vi "Multi Scan Average.vi"(8 "error in (no error)":errorcluster caption="entrée d'erreur (pas d'erreur)") -> (0 "error out":errorcluster caption="sortie d'erreur")   [LabVIEW 2019, in "Calculations.lvclass"]
uses:
  Calculations Class/Calculations.lvclass
  C:/Programmes Labview/LabScanV1A/DevicesClass/BaseDevice/BaseDevice.lvclass
  DevicesClass/BaseDevice/Accessor/GetClassEvent.vi
panel:
  out "Calculations Out.lvclass":refnum<class "Calculations.lvclass">
  in  "Calculations.lvclass":refnum<class "Calculations.lvclass">
  in  "Tab":enum32{"Description"}(tab)
  out "CalcDescription":string="Perform a running average on the selected data source. The function will average the last n data samples, where n is the \"Sample Count\" parameter provided"
  out "CalcPanelName":string="Multi Scan Average"
  in  "EditorProgQ":refnum<queue>
  in  "EditorProgQEvent":refnum<user-event>
  in  "Stop":bool
  out "Init Program":bool
  # "Multi Scan Average"
  # "this MUST be present and labeled \"Stop\""
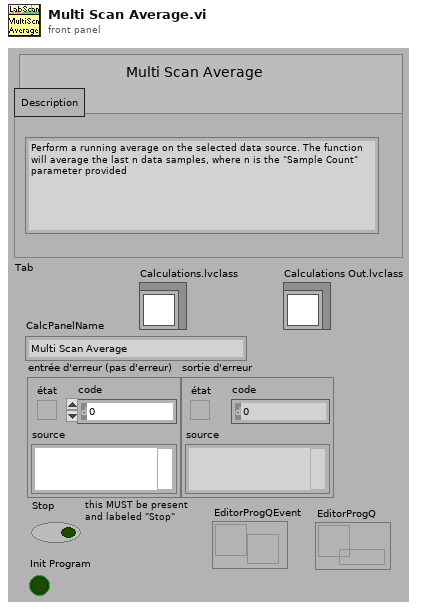
[diagram p1: front panel]
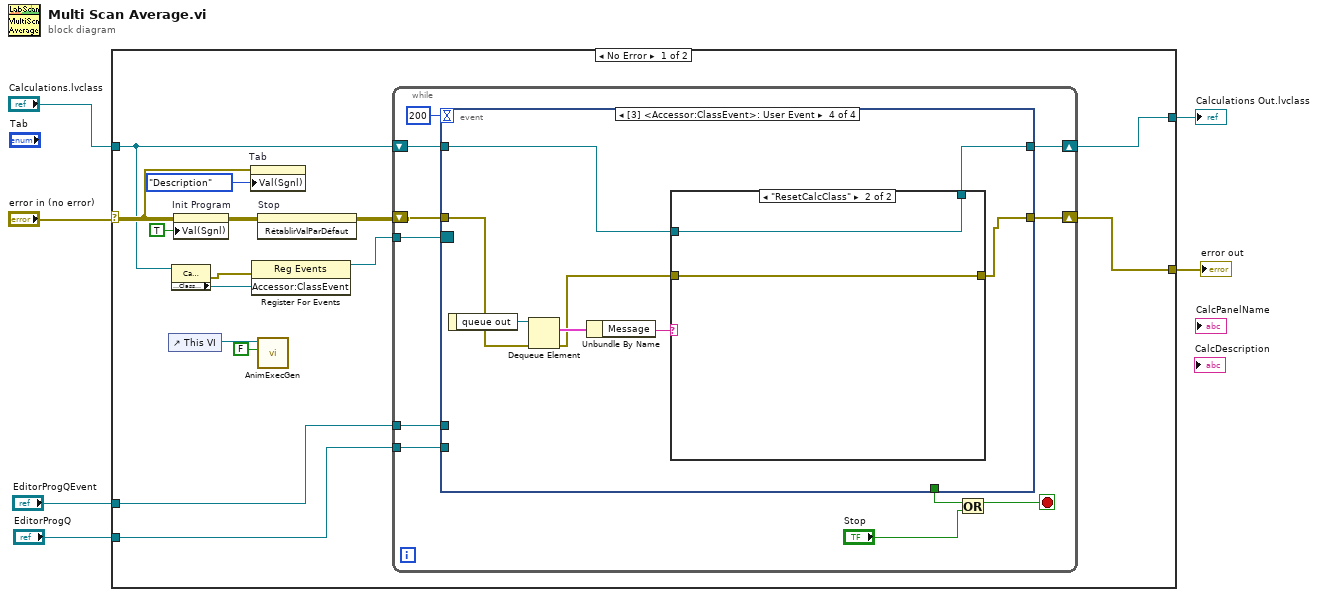
[diagram p0: block diagram]
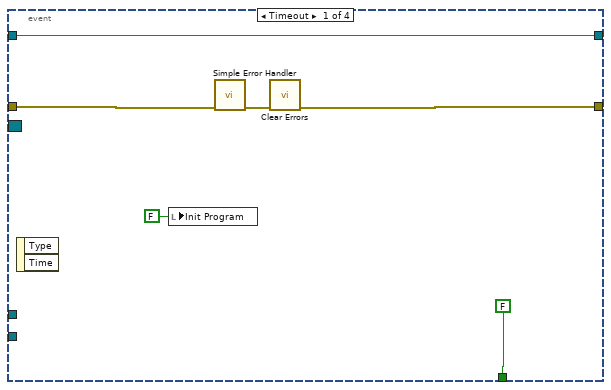
[diagram p2: hidden frame]
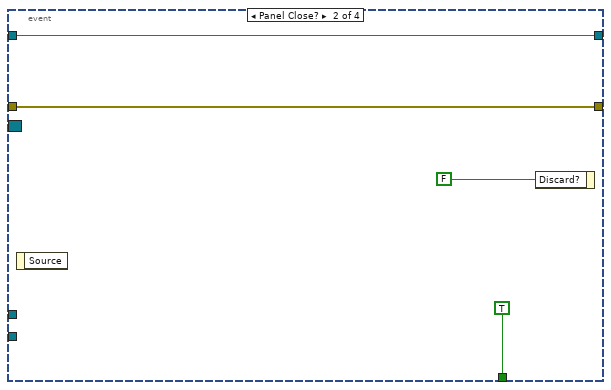
[diagram p3: hidden frame]
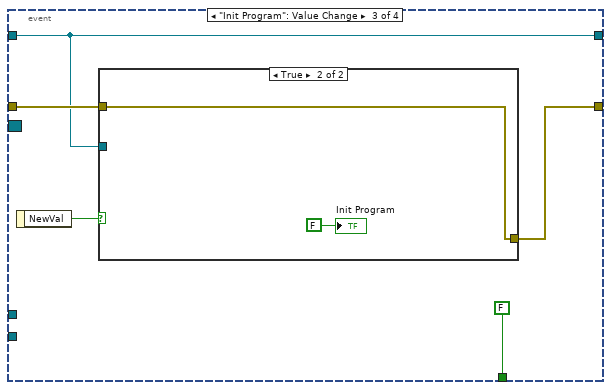
[diagram p4: hidden frame]
diagram:
  n1 = case shown="No Error" "error in (no error)" {
    selector: "error in (no error)" -> [w7 w64]
    tunnel: [w21 w64] -> w5
    tunnel: "EditorProgQEvent" -> [w15 _]
    tunnel: "EditorProgQ" -> [w14 _]
    tunnel: "Calculations.lvclass" -> [w9 w63]
    tunnel: [w13 w63] -> w1
    frame No Error {
      n2 = control-ref of="This VI"() -> (w16:refnum<vi>)
      n3 = property class="Calculations.lvclass"(reference=w9) -> (error out=w12:errorcluster, "Accessor:ClassEvent"=w11:refnum<user-event>)  [unwired: 1 in, 1 out]
      n4 = property on="Init Program" class="Bool (strict)"(error in=w7, "Val(Sgnl)"=TRUE ("Valeur (Signalisation)")) -> (error out=w19:errorcluster)  [unwired: 1 in, 1 out]
      n5 = property on="Tab" class="Onglet (strict)"(error in=w7, "Val(Sgnl)"=enum32{"Description"}."Description" ("Valeur (Signalisation)")) -> ()  [unwired: 1 in, 2 out]
      n6 = register-events(error in=w12, w11) -> (reference out=w10:refnum<event-registration>)  [unwired: 1 in, 1 out]
      n7 = invoke on="Stop" class="Bool (strict)" method="RétablirValParDéfaut"(error in=w19) -> (error out=w18:errorcluster)  [unwired: 2 in, 2 out]
      n8 = call <userlib>:"AnimExecGen.vi"("Animer l'exécution ?"=FALSE, "ViRef"=w16) -> ()  [unwired: 9 in, 1 out]
      n9 = while {
        shift-right: [w30] -> w21
        shift-left: w18 -> [w31]
        tunnel: w15 -> [w26]
        tunnel: w14 -> [w25]
        shift-right: [w23] -> w13
        shift-left: w9 -> [w24]
        tunnel: w10 -> [w22]
        stop <- w28 stop-if-true
        n10 = event shown="[3] <Accessor:ClassEvent>: User Event" {
          selector: w22 -> [_ _ _ _]
          dyn-events: _ -> [_ _ _ _]
          timeout: 200 -> [_ _ _ _]
          tunnel: w31 -> [w37 w40 w46 w52]
          tunnel: [w35 w40 w45 w54] -> w30
          tunnel: [FALSE TRUE FALSE _] -> w29
          tunnel: w26 -> [_ _ _ _]
          tunnel: w25 -> [_ _ _ _]
          tunnel: w24 -> [w33 w39 w43 w55]
          tunnel: [w33 w39 w43 w56] -> w23
          event Timeout {
            n11 = event-data() -> ()  [unwired: 1 in, 2 out]
            n12 = local write "Init Program"(FALSE ("Init Program")) -> ()
            n13 = call <vilib>:"Simple Error Handler.vi"("error in (no error)"=w37) -> ("error out"=w36:errorcluster)  [unwired: 4 in, 4 out]
            n14 = call <vilib>:"Clear Errors.vi"("error in (no error)"=w36) -> ("error out"=w35:errorcluster)  [unwired: 5 in, 1 out]
          }
          event Panel Close? {
            n15 = event-data() -> ()  [unwired: 1 in, 1 out]
            n16 = event-data("Discard?"=FALSE ("Rejeter ?")) -> ()  [unwired: 1 in, 1 out]
          }
          event "Init Program": Value Change {
            n17 = event-data() -> ("NewVal"=w47:bool)  [unwired: 1 in]
            n18 = case shown="True" w47 {
              tunnel: w46 -> [w48 w49]
              tunnel: [w48 w49] -> w45
              tunnel: w43 -> [_ _]
              frame False {
              }
              frame True {
                "Init Program" <- FALSE
              }
            }
          }
          event User Event {
            n19 = event-data() -> ("queue out"=w58:refnum<queue>)  [unwired: 1 in]
            n20 = Dequeue Element(queue=w58, error in (no error)=w52) -> (element=w53:cluster{"Message":string, "Data":variant, i32}, error out=w51:errorcluster)  [unwired: 1 in, 2 out]
            n21 = Unbundle By Name(w53) -> ("Message"=w57:string)
            n22 = case shown="\"ResetCalcClass\"" w57 {
              tunnel: [w60 w61] -> w56
              tunnel: w55 -> [w60 w61]
              tunnel: [w59 w62] -> w54
              tunnel: w51 -> [w59 w62]
              frame Default {
              }
              frame "ResetCalcClass" {
              }
            }
          }
        }
        n23 = Or(x=w29, y="Stop") -> (x .or. y?=w28:bool)
      }
    }
    frame Error {
    }
  }
  "error out" <- w5
  "Calculations Out.lvclass" <- w1
